vi "Dashboard Main.vi"() -> ()   [LabVIEW 2015]
uses:
  <vilib>/Utility/miscctls.llb/LVRowAndColumnTypeDef.ctl
  <vilib>/event_ctls.llb/eventvkey.ctl
  <vilib>/Rock Robotics/WPI/Dashboard/WPI_DashboardLogging Global.vi
  <vilib>/Rock Robotics/Network Tables/NT Read Numeric Array.vi
  <vilib>/Rock Robotics/Network Tables/NT Read Boolean.vi
  <vilib>/Rock Robotics/Network Tables/NT Write Boolean.vi
  <vilib>/Utility/config.llb/Write Key (String).vi
  <vilib>/Utility/config.llb/Write Key (I32).vi
  <vilib>/Utility/config.llb/NI_LVConfig.lvlib
panel:
  in  "TCP":refnum<k5>
  in  "Rec Mode":enum32{"Stop", "Record", "Playback"}(radio)
  in  "Vision":u16(ring) items=["Camera Off", "USB Camera SW", "USB Camera HW", "IP Camera"]
  out "Camera IP":string
  out "Image Message":string="Timeout in Camera Communications"
  in  "Dashboard Tab":T1(tab)
  in  "Select Auto":string(combo)
  out "NT Connection":bool
  in  "Camera Settings":T2={"Frame Rate"=30, "Compression"=30, "Size"=1} {"Frame Rate" scale=1.0..30.0; "Size" items=["640x480", "320x240", "160x120"]}
  out "MotorChart R":cluster{"Numeric":dbl, "Numeric":dbl}(graph)
  out "MotorChart L":T3(graph)
  out "MotorSliders R":cluster{"MotorSlide1":dbl, "MotorSlide2":dbl} {"MotorSlide2" scale=-1.0..1.0 scale format="%#_2e"; "MotorSlide1" scale=-1.0..1.0 scale format="%#_2e"}
  out "MotorSliders L":T4 {"MotorSlide4 2" scale=0.0..14.0 scale format="%#_2e"; "MotorSlide2" scale=-1.0..1.0 scale format="%#_2e"; "MotorSlide1" scale=-1.0..1.0 scale format="%#_2e"}
  out "Gyro":dbl(knob) scale=0.0..360.0
  out "JS1 Z":dbl(slide) scale=-1.0..1.0 scale format="%#_2e"
  out "JS1 Graph":cluster{"X":dbl, "Y":dbl}[](graph)
  out "JS1 Buttons":T5
  out "JS2 Z":dbl(slide) scale=-1.0..1.0 scale format="%#_2e"
  out "JS2 Graph":cluster{"X":dbl, "Y":dbl}[](graph)
  out "JS2 Buttons":T5
  out "Mode":T6(ring)=enum."Auto Disabled"
  in  "DB Camera Config":bool
  out "fps":dbl format="%#.1g"
  out "Mbps":dbl format="%#.1g"
  out "Mbps LED":bool
  in  "DB/String 9":string
  in  "DB/String 8":string
  in  "DB/String 7":string
  in  "DB/String 6":string
  in  "DB/String 5":string
  in  "DB/String 4":string
  in  "DB/String 3":string
  in  "DB/String 2":string
  in  "DB/String 1":string
  in  "DB/String 0":string
  in  "DB/Slider 0":dbl(slide) scale=0.0..5.0
  in  "DB/Slider 1":dbl(slide) scale=0.0..5.0
  in  "DB/Slider 2":dbl(slide) scale=0.0..5.0
  in  "DB/Slider 3":dbl(slide) scale=0.0..5.0
  out "DB/LED 3":bool
  out "DB/LED 2":bool
  out "DB/LED 1":bool
  out "DB/LED 0":bool
  in  "DB/Button 3":bool
  in  "DB/Button 2":bool
  in  "DB/Button 1":bool
  in  "DB/Button 0":bool caption="New Name"
  in  "Lower Shoot On Start of Auto":bool=TRUE
  in  "Auto Mode \nSelector":dbl
  out "?":dbl(slide)=88.0 scale=78.0..98.0
  out "POT Online?":bool
  out "?":dbl(knob)=87.99999517335185 scale=78.0..98.0
  out "True Solid Value":dbl=88.0
  out "POT Sensor":dbl(knob)=88.0000526149156 scale=78.0..98.0
  out "Low Sensor":bool=TRUE
  out "High Sensor":bool=TRUE
  in  "Test Slider":dbl(slide) scale=0.0..100.0 scale format="%#_3g"
  in  "On/Off":bool caption="Solenoid"
  in  "Test Name":u16(ring) items=["Select the test to run..."]
  in  "Test Tree":string(tree)
  in  "Motor":cluster{"Value":dbl, "Enable":bool} {"Value" scale=-1.0..1.0 scale format="%#_3g"}
  out "Progress":T7 {"Test Progress" scale=0.0..100.0}
  in  "Rev/Fwd":cluster{"Forward":bool, "Reverse":bool}
  in  "Test Ring":u16(ring) items=["Monochrome", "Color"]
  out "Cmd Status":string
  in  "Execute Command":bool
  in  "Command Params":string[][](table)
  in  "Command Selection":i32(listbox)
  in  "CheckList":i32(listbox)
  out "Tree":string(tree)
  out "Camera Image":T8(plugin-control)
  out "Background":bool
  # "Left"
  # "Front"
  # "Right"
  # "Battery"
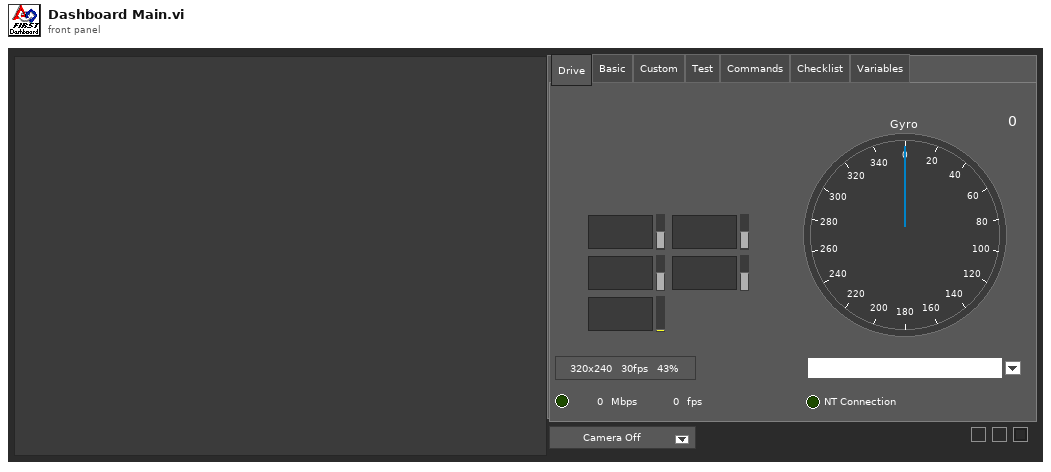
[diagram p1: front panel]
types:
  T1 = enum32{"Drive", "Basic", "Custom", "Test", "Commands", "Checklist", "Variables"}
  T2 = cluster{"Frame Rate":i32, "Compression":i32, "Size":u16}
  T3 = cluster{"Numeric":dbl, "Numeric":dbl, "Battery V":dbl}
  T4 = cluster{"MotorSlide1":dbl, "MotorSlide2":dbl, "MotorSlide4 2":dbl}
  T5 = cluster{bool, bool, bool, bool, bool, bool, bool, bool, bool, bool, bool, bool}
  T6 = enum8{"Tele-Op Disabled", "Tele-Op Enabled", "Auto Disabled", "Auto Enabled", "Test Disabled", "Test Enabled", "Disconnected", "No Code", "E-Stop"}
  T7 = cluster{"Test Progress":u8, "Test Progress Text":string}
  T8 = typedef "IMAQ Image.ctl" = refnum<image>
  T9 = cluster{"IDs":cluster{"RPC field ID":u16, "Unique ID":u16}, "String":string}
  T10 = enum32{"Drive", "Basic", "Custom", "Test", "Checklist", "Variables"}
  T11 = typedef "Image Type" = u32
  T12 = cluster{"Camera Image":refnum<vi>, "Dashboard Tab":refnum<vi>, "Background":refnum<vi>, "Vision":refnum<vi>, "Rec Mode":refnum<vi>, "Test Slider":refnum<vi>, "On/Off ":refnum<vi>, "Test Ring":refnum<vi>, "Rev/Fwd":refnum<vi>, "Test Name":refnum<vi>, "Motor":refnum<vi>, "Progress":refnum<vi>, "CheckList":refnum<vi>, "Tree":refnum<vi>, "Test Tree":refnum<vi>, "Command Params":refnum<vi>, "Command Selection":refnum<vi>, "Execute Command":refnum<vi>, "Cmd Status":refnum<vi>}
  T13 = cluster{"Error Strings":string, "Disable Counts":cluster{u16, u16}, "Rail Faults":cluster{u16, u16, u16}, "Robot IP":string, "DB Mode":u8, "Event Info":cluster{"Name":string, "Type":u8, "Number":u16, "Replay":u8}, "Camera Addr":string}
  T14 = cluster{"Storage":cluster{"Disk Free":u64, "RAM Block":u32, "RAM free":u32}, "CPU Utilization":cluster{"CPU % ISR":sgl, "CPU % Time Crit":sgl, "CPU % Timed Str":sgl, "CPU % High":sgl, "CPU % Above":sgl, "CPU % Normal":sgl, "CPU % Low":sgl}, "CAN":cluster{"% Bus Utilization":sgl, "Bus Off Cnt":u32, "TX_FIFO Full Cnt":u32, "Receive Error Cnt":u8, "Transmit Error Cnt":u8}, "HID":cluster{"HID Outputs":u32, "Rumble Low":u16, "Rumble High":u16}[]}
  T15 = cluster{"Status bits":cluster{"Test Mode":bool, "Autonomous":bool, "Enabled":bool, "Code Start":bool, "Brownout":bool, "Reserved 2":bool, "Reserved 3":bool, "E-Stop":bool}, "Code Trace":cluster{"Disabled":bool, "TeleOp":bool, "Auto":bool, "Test":bool}, "Controller Type":enum16{"unknown", "cRIO", "roboRio"}, "Code?":enum16{"unknown", "noCode", "code"}, "Battery V":dbl}
  T16 = cluster{"Control Bits":cluster{"TestMode":bool, "Autonomous":bool, "Enabled":bool, "FMS Present":bool, bool, bool, bool, "E-Stop":bool}, "Team Station ":u8, "Countdown":sgl, "Joystick Values":cluster{"Axes":dbl[], "Buttons":bool[], "POVs":i16[]}[]}
  T17 = cluster{"Axes":dbl[], "Buttons":bool[], "POVs":i16[]}[]
  T18 = cluster{"Axes":dbl[], "Buttons":bool[], "POVs":i16[]}
  T19 = cluster{"Buttons[0]":bool, "Buttons[1]":bool, "Buttons[2]":bool, "Buttons[3]":bool, "Buttons[4]":bool, "Buttons[5]":bool, "Buttons[6]":bool, "Buttons[7]":bool, "Buttons[8]":bool, "Buttons[9]":bool, "Buttons[10]":bool, "Buttons[11]":bool}
  T20 = typedef "NI_LVConfig.lvlib/Config Data RefNum.ctl" = refnum<k1>
  T21 = cluster{"Operation":enum16{"Update", "Clear"}, "Color Box":u32}[]
  T22 = typedef "eventvkey.ctl" = enum16{"ASCII", "Enter", "Return", "Shift", "Ctrl", "Alt", "Cmd", "Opt", "Caps", "NumLock", "Clear", "Break", "Up", "Down", "Left", "Right", "Insert", "Delete", "Home", "End", "PageUp", "PageDown", "Escape", "Help", "Pause", "ScrollLock", "F1", "F2", "F3", "F4", "F5", "F6", "F7", "F8", "F9", "F10", "F11", "F12", "F13", "F14", "F15", "F16", "F17", "F18", "F19", "F20", "F21", "F22", "F23", "F24", "Play", "VolumeUp", "VolumeDown", "Mute", "Two Byte Char"}
  T23 = cluster{"Image Size":bool, "Image Type":bool, "Pixel Value":bool, "ROI Information":bool, "Zoom Factor":bool}
  T24 = enum8{"Enabled", "Disabled", "Disabled and Grayed Out"}
  T25 = cluster{"Operation":enum16{"Update", "Clear"}, "Color Box":u32}
  T26 = typedef "LVRowAndColumnTypeDef.ctl" = cluster{"Row":i32, "Column":i32}
  T27 = cluster{"Shift":bool, "Ctrl":bool, "Alt":bool, "Cmd":bool, "Opt":bool}
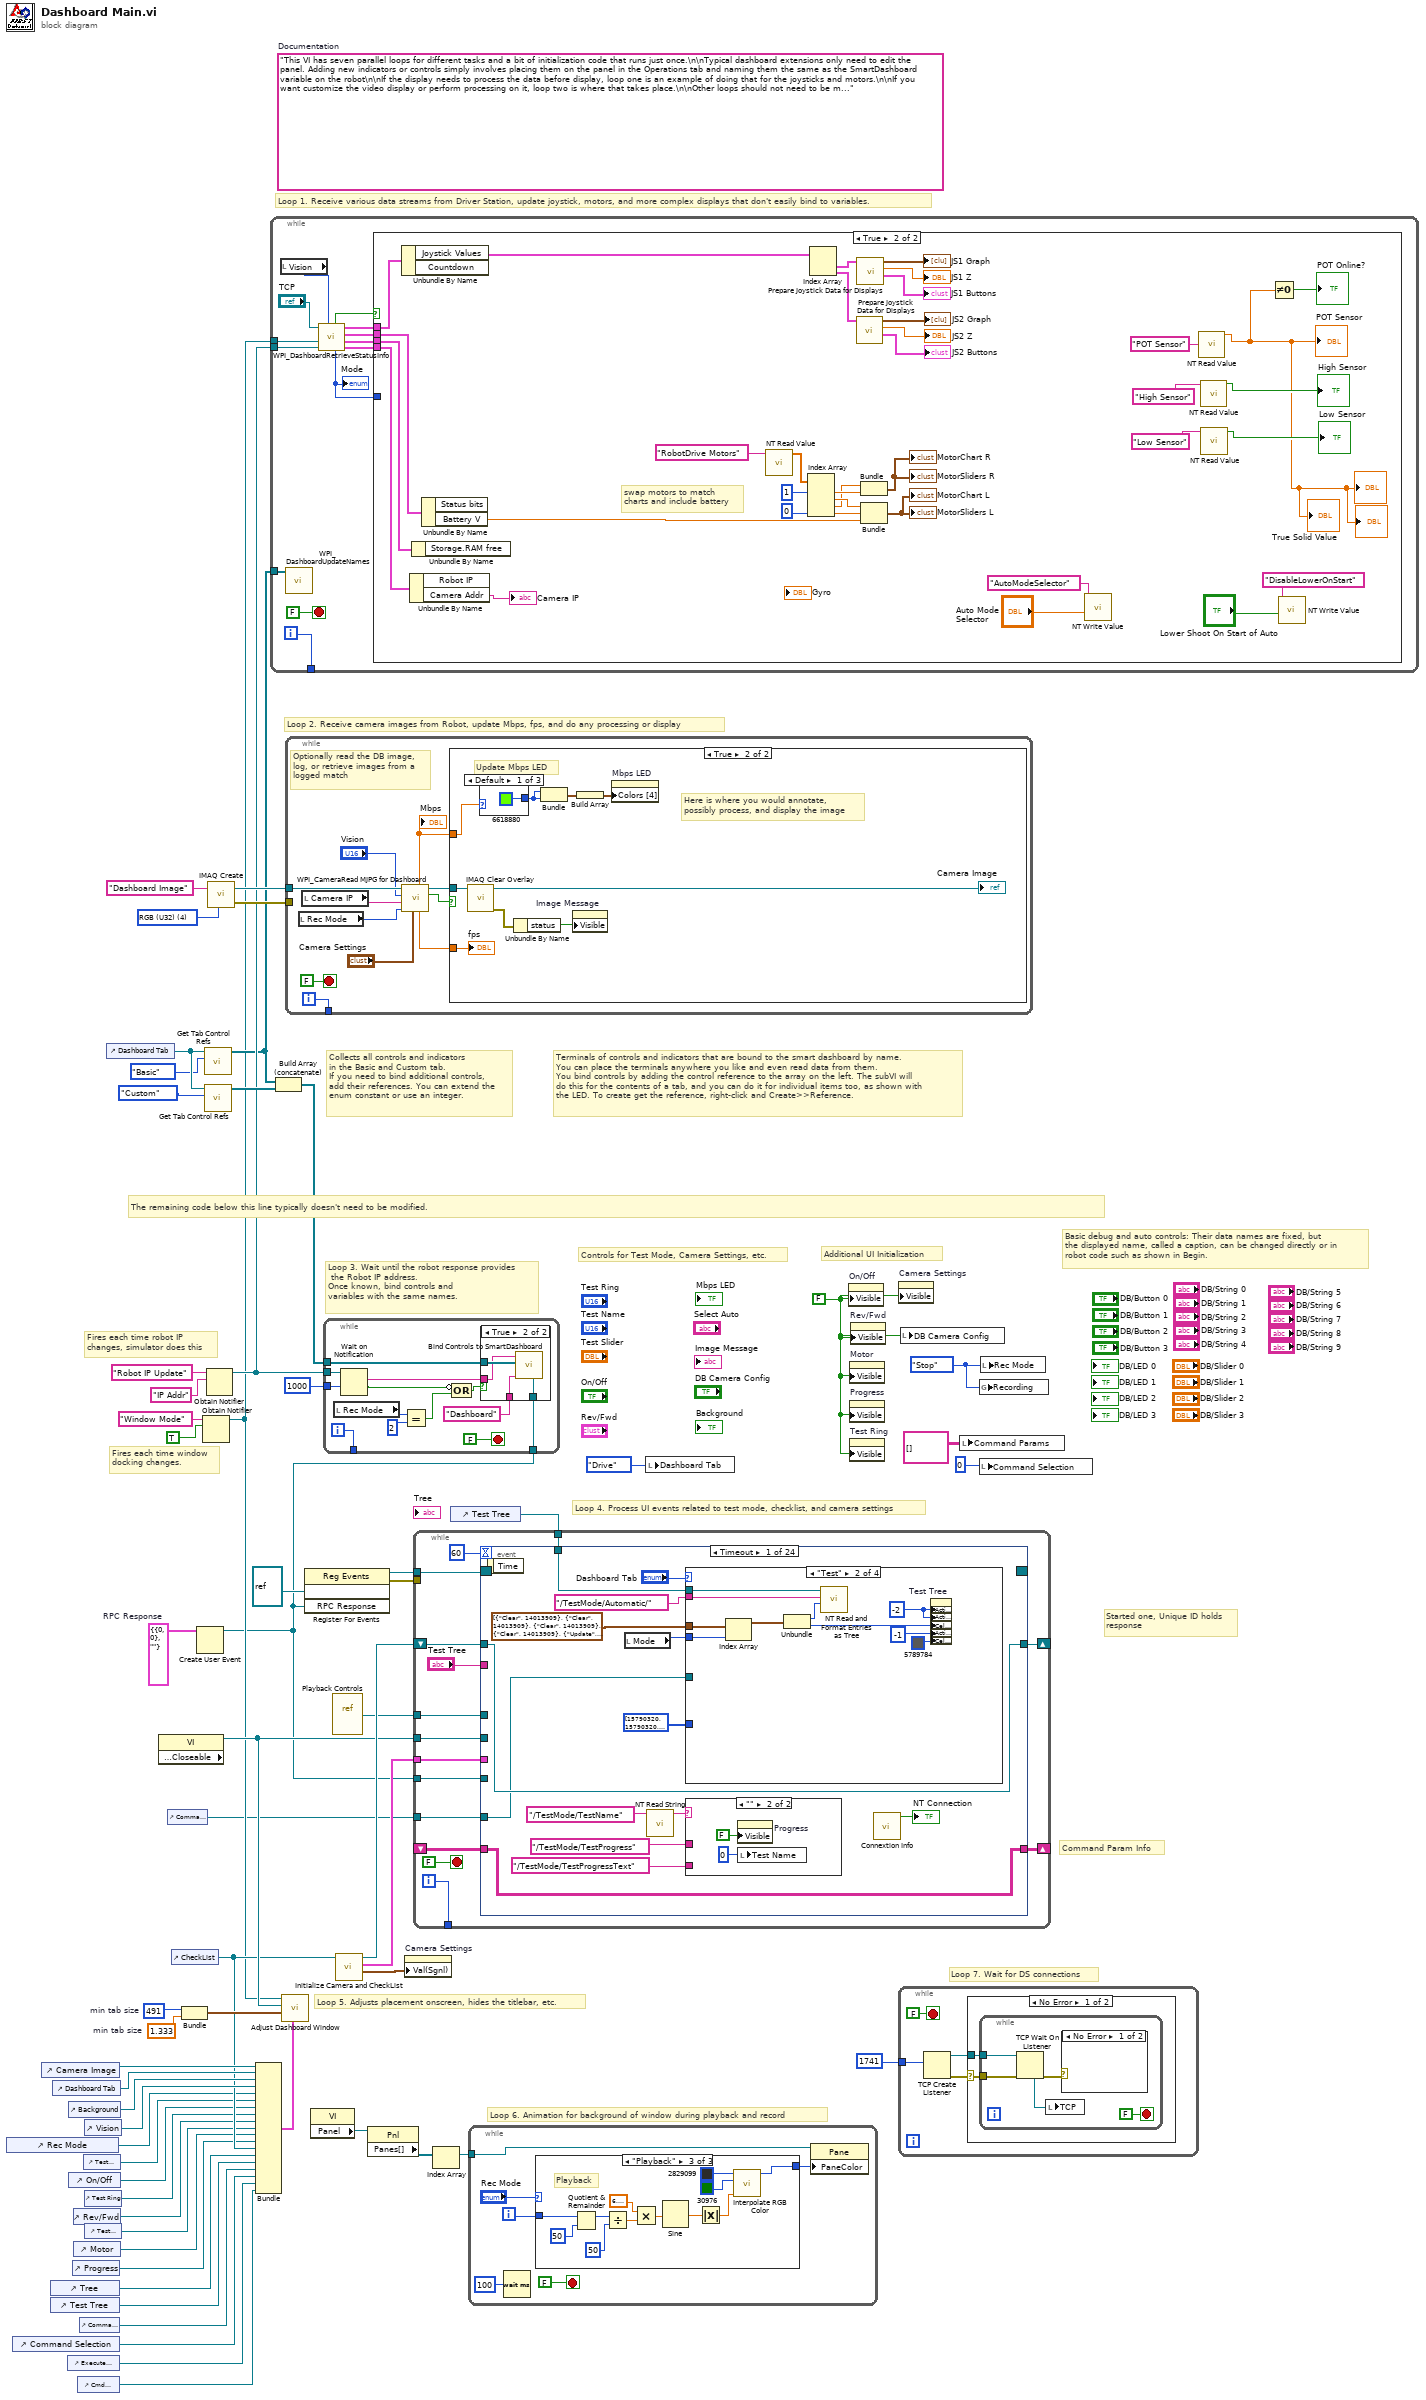
[diagram p0: block diagram]
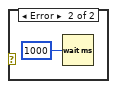
[diagram p2: hidden frame]
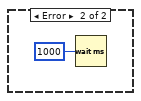
[diagram p3: hidden frame]
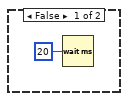
[diagram p4: hidden frame]
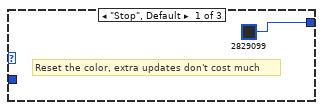
[diagram p5: hidden frame]
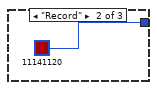
[diagram p6: hidden frame]
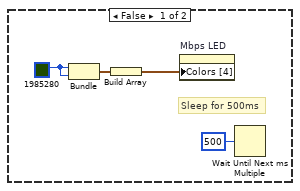
[diagram p8: hidden frame]
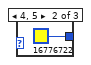
[diagram p9: hidden frame]
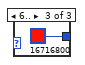
[diagram p10: hidden frame]
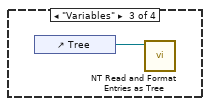
[diagram p12: hidden frame]
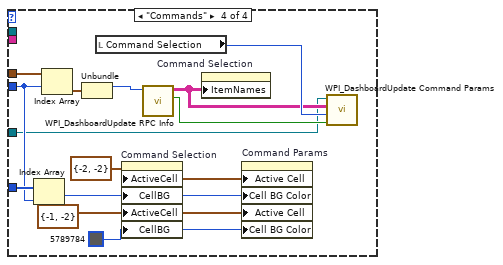
[diagram p13: hidden frame]
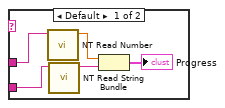
[diagram p14: hidden frame]
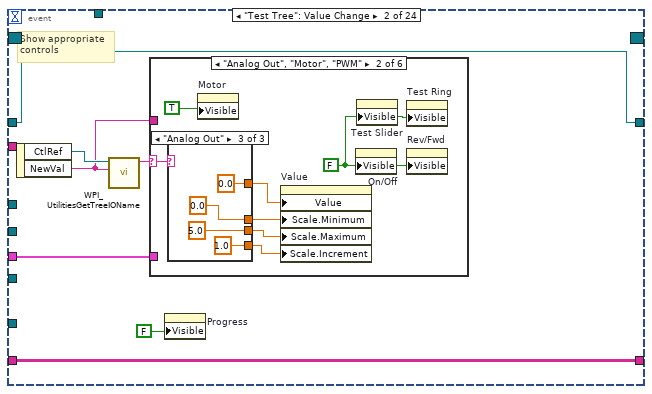
[diagram p15: hidden frame]
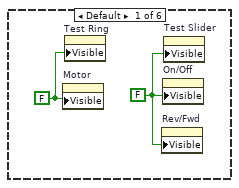
[diagram p16: hidden frame]
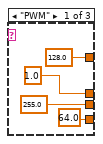
[diagram p17: hidden frame]
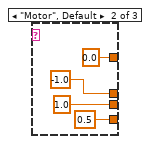
[diagram p18: hidden frame]
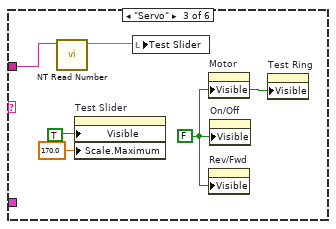
[diagram p19: hidden frame]
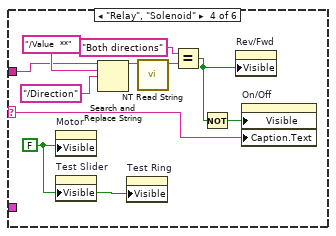
[diagram p20: hidden frame]
diagram:
  w7 = T9 {"IDs"={"RPC field ID"=0, "Unique ID"=0}, "String"=""}  # RPC Response
  w33 = 491  # min tab size
  w32 = 1.333  # min tab size
  w41 = enum32{"Stop", "Record", "Playback"}."Stop" ("Rec Mode")
  w15 = FALSE ("Visible")
  (unwired) "This VI has seven parallel loops for different tasks and a bit of initialization code that runs just once.\n\nTypical dashboard extensions only need to edit the panel. Adding new indicators or controls simply involves placing them on the panel in the Operations tab and naming them the same as the SmartDashboard variable on the robot\n\nIf the display needs to process the data before display, loop one is an example of doing that for the joysticks and motors.\n\nIf you want customize the video display or perform processing on it, loop two is where that takes place.\n\nOther loops should not need to be modified. They are pretty standard, and document the task they perform."  # Documentation
  w61 = T11 4 items=["Grayscale (U8)", "Grayscale (I16)", "Grayscale (SGL)", "Complex (CSG)", "RGB (U32)", "HSL (U32)", "RGB (U64)"] ("Image Type")
  # "Command Param Info"
  # "Started one, Unique ID holds\nresponse"
  # "Loop 7. Wait for DS connections"
  # "Basic debug and auto controls: Their data names are fixed, but\nthe displayed name, called a caption, can be changed directly or in\nrobot code such as shown in Begin."
  # "Controls for Test Mode, Camera Settings, etc."
  # "Additional UI Initialization"
  # "Loop 6. Animation for background of window during playback and record"
  # "Fires each time robot IP\nchanges, simulator does this"
  # "Fires each time window\ndocking changes."
  # "Collects all controls and indicators\nin the Basic and Custom tab.\nIf you need to bind additional controls,\nadd their references. You can extend the\nenum constant or use an integer."
  # "The remaining code below this line typically doesn't need to be modified."
  # "Loop 4. Process UI events related to test mode, checklist, and camera settings"
  # "Terminals of controls and indicators that are bound to the smart dashboard by name.\nYou can place the terminals anywhere you like and even read data from them.\nYou bind controls by adding the control reference to the array on the left. The subVI will\ndo this for the contents of a tab, and you can do it for individual items too, as shown with\nthe LED. To create get the reference, right-click and Create>>Reference."
  # "Loop 3. Wait until the robot response provides\n the Robot IP address.\nOnce known, bind controls and\nvariables with the same names."
  # "Loop 5. Adjusts placement onscreen, hides the titlebar, etc."
  # "Loop 1. Receive various data streams from Driver Station, update joystick, motors, and more complex displays that don't easily bind to variables."
  # "Loop 2. Receive camera images from Robot, update Mbps, fps, and do any processing or display"
  n1 = control-ref of="Rec Mode"() -> (w21:refnum<vi>)
  n2 = control-ref of="Command Selection"() -> (w6:refnum<vi>)
  n3 = control-ref of="Camera Image"() -> (w36:refnum<vi>)
  n4 = control-ref of="Tree"() -> (w25:refnum<vi>)
  n5 = control-ref of="Test Tree"() -> (w24:refnum<vi>)
  n6 = control-ref of="Dashboard Tab"() -> (w35:refnum<vi>)
  n7 = control-ref of="Execute Command"() -> (w8:refnum<vi>)
  n8 = control-ref of="Background"() -> (w30:refnum<vi>)
  n9 = control-ref of="On/Off"() -> (w19:refnum<vi>)
  n10 = control-ref of="Progress"() -> (w16:refnum<vi>)
  n11 = control-ref of="Rev/Fwd"() -> (w17:refnum<vi>)
  n12 = control-ref of="Motor"() -> (w22:refnum<vi>)
  n13 = control-ref of="Cmd Status"() -> (w2:refnum<vi>)
  n14 = control-ref of="Command Params"() -> (w9:refnum<vi>)
  n15 = control-ref of="Test Slider"() -> (w20:refnum<vi>)
  n16 = control-ref of="Vision"() -> (w34:refnum<vi>)
  n17 = control-ref of="Test Ring"() -> (w18:refnum<vi>)
  n18 = control-ref of="Test Name"() -> (w23:refnum<vi>)
  n19 = control-ref of="Dashboard Tab"() -> (w39:refnum<vi>)
  n20 = property class="VI" props=["Front Panel.Closeable"]() -> (reference out=w40:refnum<vi>)  [unwired: 2 in, 2 out]
  n21 = control-ref of="Command Params"() -> (w1:refnum<vi>)
  n22 = control-ref of="CheckList"() -> (w26:refnum<vi>)
  n23 = Bundle("min tab size"=w33, "min tab size"=w32) -> (w31:cluster{"min tab size":i32, "min tab size":dbl})  [unwired: 1 in]
  n24 = Create User Event(user event datatype=w7) -> (user event=w3:refnum<user-event>)  [unwired: 1 in, 1 out]
  n25 = Obtain Notifier(name (unnamed)="Window Mode", notification data type=TRUE) -> (notifier out=w12:refnum<notifier>)  [unwired: 2 in, 2 out]
  n26 = call <vilib>:"Get Tab Control Refs.vi"("Page Index"=T10."Basic" ("Dashboard Tab"), "TabControl in"=w39) -> ("ControlsOnPage"=w13:refnum<vi>[])  [unwired: 9 in]
  n27 = call <vilib>:"Get Tab Control Refs.vi"("Page Index"=T10."Custom" ("Dashboard Tab"), "TabControl in"=w39) -> ("ControlsOnPage"=w38:refnum<vi>[])  [unwired: 9 in]
  n28 = Obtain Notifier(name (unnamed)="Robot IP Update", notification data type="IP Addr" ("name (unnamed)")) -> (notifier out=w14:refnum<notifier>)  [unwired: 2 in, 2 out]
  n29 = call "IMAQ Create"("Image Name"="Dashboard Image", "Image Type"=w61) -> ("New Image"=w59:T8, "error out"=w58:errorcluster)  [unwired: 2 in, 1 out]
  n30 = Bundle("Camera Image"=w36, "Dashboard Tab"=w35, "Background"=w30, "Vision"=w34, "Rec Mode"=w21, "Test Slider"=w20, "On/Off"=w19, "Test Ring"=w18, "Rev/Fwd"=w17, "Test Name"=w23, "Motor"=w22, "Progress"=w16, "CheckList"=w26, "Tree"=w25, "Test Tree"=w24, "Command Params"=w9, "Command Selection"=w6, "Execute Command"=w8, "Cmd Status"=w2) -> (w27:T12)  [unwired: 1 in]
  n31 = while {
    tunnel: [w73] -> _
    tunnel: w14 -> [w67]
    tunnel: w13 -> [w66]
    tunnel: w12 -> [w62]
    i -> [w73]
    stop <- FALSE stop-if-true
    n32 = local read "Vision"() -> (w64:u16)
    n33 = call <vilib>:"WPI_DashboardUpdateNames.vi"("Controls on Tab"=w66) -> ()  [unwired: 11 in]
    n34 = call <vilib>:"WPI_DashboardRetrieveStatusInfo.vi"("Vision"=w64, "Binding Refnum"=w67, "Window Mode Notifier"=w62, "TCP Cnx"="TCP") -> ("Power and Errors"=w68:T13, "Robot Metrics"=w71:T14, "Status Info"=w72:T15, "Control Info"=w69:T16, "Robot Mode"=w65:T6, "Process?"=w70:bool)  [unwired: 2 in]
    "Mode" <- w65
    n35 = case shown="True" w70 {
      tunnel: w72 -> [_ w111]
      tunnel: w71 -> [_ w110]
      tunnel: w69 -> [_ w109]
      tunnel: w68 -> [_ w108]
      tunnel: w65 -> [_ _]
      frame False {
        n36 = Wait (ms)(milliseconds to wait=u32 20) -> ()  [unwired: 1 out]
      }
      frame True {
        # "swap motors to match\ncharts and include battery"
        n37 = Unbundle By Name(w109) -> ("Joystick Values"=w98:T17)  [unwired: 1 out]
        n38 = Unbundle By Name(w108) -> ("Camera Addr"=→"Camera IP":string)  [unwired: 1 out]
        n39 = Unbundle By Name(w110) -> ()  [unwired: 1 out]
        n40 = Unbundle By Name(w111) -> ("Battery V"=w99:dbl)  [unwired: 1 out]
        n41 = call-poly <vilib>:"NT Read Value.vi"("Name"="RobotDrive Motors") -> ("Numeric Array"=w87:dbl[])  [unwired: 9 in, 1 out]
        n42 = Index Array(array=w87, index #1=1, index #4=0) -> (element #1=w103:dbl, element #2=w104:dbl, element #3=w102:dbl, element #4=w107:dbl)  [unwired: 2 in]
        n43 = Index Array(array=w98) -> (element #1=w97:T18, element #2=w92:T18)  [unwired: 2 in]
        n44 = call "Prepare Joystick Data for Displays.vi"("Joystick Values"=w92) -> ("Buttons"=→"JS2 Buttons":T19, "Z Axis"=→"JS2 Z":dbl, "Cartesian Data"=→"JS2 Graph":cluster{"X axis":dbl, "X axis":dbl}[])  [unwired: 8 in]
        n45 = call "Prepare Joystick Data for Displays.vi"("Joystick Values"=w97) -> ("Buttons"=→"JS1 Buttons":T19, "Z Axis"=→"JS1 Z":dbl, "Cartesian Data"=→"JS1 Graph":cluster{"X axis":dbl, "X axis":dbl}[])  [unwired: 8 in]
        n46 = Bundle("Numeric"=w102, "Numeric"=w103) -> (→"MotorChart R" →"MotorSliders R":cluster{"Numeric":dbl, "Numeric":dbl})  [unwired: 1 in]
        n47 = Bundle("Numeric"=w104, "Numeric"=w107, "Battery V"=w99) -> (→"MotorChart L" →"MotorSliders L":T3)  [unwired: 1 in]
        n48 = call-poly <vilib>:"NT Write Value.vi"("Numeric"="Auto Mode \nSelector", "Name"="AutoModeSelector") -> ()  [unwired: 9 in, 1 out]
        n49 = call-poly <vilib>:"NT Read Value.vi"("Name"="POT Sensor") -> ("Numeric"=w76:dbl)  [unwired: 9 in, 1 out]
        "POT Sensor" <- w76
        "True Solid Value" <- w76
        "?" <- w76
        "?" <- w76
        n50 = call-poly <vilib>:"NT Read Value.vi"("Name"="High Sensor") -> ("Boolean"=→"High Sensor":bool)  [unwired: 9 in, 1 out]
        n51 = call-poly <vilib>:"NT Read Value.vi"("Name"="Low Sensor") -> ("Boolean"=→"Low Sensor":bool)  [unwired: 9 in, 1 out]
        n52 = Not Equal To 0?(x=w76) -> (x != 0?=→"POT Online?":bool)
        n53 = call-poly <vilib>:"NT Write Value.vi"("Boolean"="Lower Shoot On Start of Auto", "Name"="DisableLowerOnStart") -> ()  [unwired: 9 in, 1 out]
      }
    }
  }
  n54 = Build Array (concatenate)(w13, w38) -> (w37:refnum<vi>[])
  n55 = call "Adjust Dashboard Window.vi"("Sizing Refnums"=w27, "Size Constraints"=w31, "VI"=w40, "WIn Mode"=w12) -> ()  [unwired: 8 in]
  n56 = while {
    tunnel: w59 -> [w120]
    tunnel: w58 -> [_]
    tunnel: [w121] -> _
    i -> [w121]
    stop <- FALSE stop-if-true
    # "Optionally read the DB image,\nlog, or retrieve images from a\nlogged match"
    n57 = local read "Rec Mode"() -> (w115:enum32{"Stop", "Record", "Playback"})
    n58 = local read "Camera IP"() -> (w113:string)
    n59 = call <vilib>:"WPI_CameraRead MJPG for Dashboard.vi"("Camera Settings"="Camera Settings", "Rec Mode"=w115, "Camera IP"=w113, "Camera Mode"="Vision", "Refnum in"=w120) -> ("Active"=w118:bool, "Refnum out"=w119:T8, "FPS"=w117:dbl, "Bandwidth (Mbps)"=w112:dbl)  [unwired: 3 in]
    "Mbps" <- w112
    n60 = case shown="True" w118 {
      tunnel: w119 -> [_ w130]
      tunnel: w112 -> [_ w129]
      tunnel: w117 -> [_ w127]
      frame False {
        w123 = u32 1985280 ("Color Box")
        # "Sleep for 500ms"
        n61 = Bundle("Color Box"=w123, "Color Box"=w123) -> (w125:cluster{"Color Box":u32, "Color Box":u32})  [unwired: 1 out]
        n62 = Build Array(w125) -> (w124:cluster{"Color Box":u32, "Color Box":u32}[])
        n63 = property on="Mbps LED" class="Bool (strict)"("Colors [4]"=w124) -> ()  [unwired: 2 in, 2 out]
        n64 = Wait Until Next ms Multiple(millisecond multiple=u32 500) -> ()  [unwired: 1 out]
      }
      frame True {
        # "Here is where you would annotate,\npossibly process, and display the image"
        # "Update Mbps LED"
        n65 = call "IMAQ Clear Overlay"("Image"=w130) -> ("error out"=w134:errorcluster, "Image Out"=→"Camera Image":T8)  [unwired: 2 in, 7 out]
        n66 = case shown="Default" w129 {
          tunnel: [u32 6618880 ("Color Box") u32 16776722 ("Color Box") u32 16716800 ("Color Box")] -> w131
          frame Default {
          }
          frame 4, 5 {
          }
          frame 6.. {
          }
        }
        n67 = Unbundle By Name(w134) -> ("status"=w135:bool)
        n68 = Bundle("Color Box"=w131, "Color Box"=w131) -> (w133:cluster{"Color Box":u32, "Color Box":u32})  [unwired: 1 out]
        n69 = property on="Image Message" class="Str"("Visible"=w135) -> ()  [unwired: 2 in, 2 out]
        n70 = Build Array(w133) -> (w132:cluster{"Color Box":u32, "Color Box":u32}[])
        n71 = property on="Mbps LED" class="Bool (strict)"("Colors [4]"=w132) -> ()  [unwired: 2 in, 2 out]
        "fps" <- w127
      }
    }
  }
  n72 = register-events(refnum<vi> refnum, w3) -> (reference out=w45:refnum<event-registration>, error out=w44:errorcluster)  [unwired: 2 in]
  n73 = property class="VI"() -> ("Panel"=w48:refnum<vi>)  [unwired: 2 in, 2 out]
  n74 = while {
    tunnel: w37 -> [w151]
    tunnel: w14 -> [w149]
    tunnel: [w147] -> _
    tunnel: u32 1000 ("milliseconds to wait") -> [w146]
    tunnel: w3 -> [w139]
    i -> [w147]
    stop <- FALSE stop-if-true
    n75 = local read "Rec Mode"() -> (w142:enum32{"Stop", "Record", "Playback"})
    n76 = Wait on Notification(notifier=w149, timeout in ms (-1)=w146) -> (notification=w148:string, timed out?=w144:bool)  [unwired: 2 in, 2 out]
    n77 = Equal?(x=w142, y=u16 2 ("Rec Mode")) -> (x = y?=w143:bool)
    n78 = Compound Arithmetic op=OR(invert w144, w143) -> (w145:bool)
    n79 = case shown="True" w145 {
      tunnel: w151 -> [_ w155]
      tunnel: w148 -> [_ w154]
      tunnel: "Dashboard" -> [_ w153]
      tunnel: w139 -> [_ w152]
      frame False {
      }
      frame True {
        n80 = call <vilib>:"Bind Controls to SmartDashboard.vi"("RPC ref"=w152, "Client Name"=w153, "Bound Control Refs"=w155, "Server IP Address"=w154) -> ()  [unwired: 8 in]
      }
    }
  }
  n81 = vi-ref "Playback Controls.vi"() -> (w46:refnum<vi>)
  n82 = call "Initialize Camera and CheckList.vi"("ListBox in"=w26) -> ("Cluster"=w52:cluster{"value":i32, "value":i32, "index":i32}, "Array"=w53:cluster{string[]}[], "File Refnum"=w51:T20)  [unwired: 8 in]
  n83 = property class="Pnl"(reference=w48) -> ("Panes[]"=w49:refnum<vi>[])  [unwired: 1 in, 2 out]
  n84 = property on="Camera Settings" class="Clust (strict)"("Val(Sgnl)"=w52) -> ()  [unwired: 2 in, 2 out]
  n85 = Index Array(array=w49) -> (element=w47:refnum<vi>)  [unwired: 1 in]
  n86 = control-ref of="Test Tree"() -> (w50:refnum<vi>)
  n87 = while {
    tunnel: w53 -> [w167]
    shift-right: [w166] -> _
    shift-left: w51 -> [w165]
    tunnel: [w164] -> _
    tunnel: w50 -> [w163]
    tunnel: w46 -> [w162]
    tunnel: w45 -> [w161]
    tunnel: w44 -> [_]
    tunnel: w40 -> [w160]
    tunnel: w3 -> [w159]
    tunnel: w1 -> [w158]
    shift-right: [w157] -> _
    shift-left: _ -> [w156]
    i -> [w164]
    stop <- FALSE stop-if-true
    n88 = event shown="[0] Timeout" {
      selector: w161 -> [_ _ _ _ _ _ _ _ _ _ _ _ _ _ _ _ _ _ _ _ _ _ _ _]
      dyn-events: [_ _ _ _ _ _ _ _ _ _ _ _ _ _ _ _ _ _ w476 _ _ _ _ _] -> _
      timeout: u32 60 ("milliseconds to wait") -> [_ _ _ _ _ _ _ _ _ _ _ _ _ _ _ _ _ _ _ _ _ _ _ _]
      tunnel: w163 -> [w180 _ _ _ _ _ _ _ _ _ _ _ _ _ _ _ _ _ _ _ _ _ _ _]
      tunnel: "Test Tree" -> [_ _ _ _ _ _ _ _ _ _ _ _ _ w439 w448 w451 w456 w465 _ _ _ _ _ _]
      tunnel: w167 -> [_ w218 _ _ _ _ _ _ _ _ _ w401 w432 _ _ _ _ _ _ _ _ _ _ _]
      tunnel: [w177 w217 w321 w327 w337 w341 w347 w359 w367 w373 w386 w400 w425 w438 w446 w450 w455 w464 w478 w494 w496 w504 w515 w520] -> w166
      tunnel: w165 -> [w177 w217 w321 w327 w337 w341 w347 w359 w367 w373 w386 w399 w425 w438 w446 w450 w455 w464 w478 w494 w496 w504 w515 w520]
      tunnel: w162 -> [_ _ _ _ _ _ _ _ _ _ _ _ _ _ _ _ _ _ w479 _ w499 _ _ _]
      tunnel: w160 -> [_ _ _ _ _ _ _ _ _ _ _ _ _ _ _ _ _ _ w474 _ _ _ _ _]
      tunnel: w159 -> [_ _ _ _ _ _ _ _ _ _ _ _ _ _ _ _ _ _ w470 _ _ _ _ _]
      tunnel: w158 -> [w172 _ _ _ _ _ w345 _ _ _ _ _ _ _ _ _ _ _ _ _ _ _ _ _]
      tunnel: [w171 w216 w320 w326 w336 w342 w343 w353 w364 w372 w385 w398 w424 w437 w445 w449 w454 w463 w469 w492 w495 w500 w508 w521] -> w157
      tunnel: w156 -> [w171 w216 w320 w326 w336 w342 w343 _ _ w372 w385 w398 w424 w437 w445 w449 w454 w463 w469 w492 w495 w500 w508 w521]
      event Timeout {
        n89 = event-data() -> ()  [unwired: 1 in, 1 out]
        n90 = local read "Mode"() -> (w174:T6)
        n91 = call <vilib>:"NT Read String.vi"("Name"="/TestMode/TestName") -> ("String"=w183:string)  [unwired: 9 in, 1 out]
        n92 = case shown="\"Test\"" "Dashboard Tab" {
          tunnel: w180 -> [_ w194 _ _]
          tunnel: "/TestMode/Automatic/" ("Name Pattern") -> [_ w193 _ _]
          tunnel: T21 [{"Operation"=enum."Clear", "Color Box"=14013909}, {"Operation"=enum."Clear", "Color Box"=14013909}, {"Operation"=enum."Clear", "Color Box"=14013909}, {"Operation"=enum."Clear", "Color Box"=14013909}, {"Operation"=enum."Update", "Color Box"=14013909}, {"Operation"=enum."Update", "Color Box"=16777215}, {"Operation"=enum."Clear", "Color Box"=14013909}, {"Operation"=enum."Clear", "Color Box"=14013909}, {"Operation"=enum."Clear", "Color Box"=14013909}] -> [_ w186 _ w203]
          tunnel: w174 -> [_ w185 _ w202]
          tunnel: u32[] [15790320, 15790320, 15790320, 15790320, 16777215, 16777215, 15790320, 15790320, 15790320] -> [_ _ _ w208]
          tunnel: w172 -> [_ _ _ w196]
          frame "Custom", Default {
          }
          frame "Test" {
            w192 = -2 ("Active Item:Row Number")
            n93 = Index Array(array=w186, index=w185) -> (element=w187:T25)
            n94 = Unbundle(w187) -> ("Operation"=w188:enum16{"Update", "Clear"}, "Color Box"=w189:u32)
            n95 = call <vilib>:"NT Read and Format Entries as Tree.vi"("Operation"=w188, "Name Pattern"=w193, "Tree Refnum"=w194) -> ()  [unwired: 7 in, 2 out]
            n96 = property on="Test Tree" class="Tree (strict)"("Active Item Row Number"=w192, "ActiveColNum"=w192, "CellBG"=w189, "Active Item Row Number"=-1 ("Active Item:Row Number"), "CellBG"=u32 5789784 ("Color Box")) -> ()  [unwired: 2 in, 2 out]
          }
          frame "Variables" {
            n97 = control-ref of="Tree"() -> (w195:refnum<vi>)
            n98 = call <vilib>:"NT Read and Format Entries as Tree.vi"("Tree Refnum"=w195) -> ()  [unwired: 9 in, 2 out]
          }
          frame "Commands" {
            w204 = u32 5789784 ("Color Box")
            w205 = T26 {"Row"=-1, "Column"=-2} ("Active Cell:Active Cell")
            w207 = T26 {"Row"=-2, "Column"=-2} ("Active Cell:Active Cell")
            n99 = Index Array(array=w208, index=w202) -> (element=w206:u32)
            n100 = Index Array(array=w203, index=w202) -> (element=w201:T25)
            n101 = Unbundle(w201) -> ("Operation"=w200:enum16{"Update", "Clear"})  [unwired: 1 out]
            n102 = local read "Command Selection"() -> (w199:i32)
            n103 = property on="Command Selection" class="MCListbox (strict)"("ActiveCell"=w207, "CellBG"=w206, "ActiveCell"=w205, "CellBG"=w204) -> ()  [unwired: 2 in, 2 out]
            n104 = call <vilib>:"WPI_DashboardUpdate RPC Info.vi"("Operation"=w200) -> ("update"=w198:bool, "commands"=w197:string[][])  [unwired: 9 in]
            n105 = property on="Command Selection" class="MCListbox (strict)"("ItemNames"=w197) -> ()  [unwired: 2 in, 2 out]
            n106 = property on="Command Params" class="Tbl (strict)"("Active Cell"=w207, "Cell BG Color"=w206, "Active Cell"=w205, "Cell BG Color"=w204) -> ()  [unwired: 2 in, 2 out]
            n107 = call <vilib>:"WPI_DashboardUpdate Command Params.vi"("Update"=w198, "NewVal"=w199, "Commands"=w197, "Param Tbl"=w196) -> ()  [unwired: 7 in, 1 out]
          }
        }
        n108 = case shown="\"\"" w183 {
          tunnel: "/TestMode/TestProgress" ("Name") -> [w210 _]
          tunnel: "/TestMode/TestProgressText" ("Name") -> [w209 _]
          frame Default {
            n109 = call <vilib>:"NT Read Number.vi"("Name"=w210) -> ("Numeric"=w211:dbl)  [unwired: 9 in, 1 out]
            n110 = call <vilib>:"NT Read String.vi"("Name"=w209) -> ("String"=w212:string)  [unwired: 9 in, 1 out]
            n111 = Bundle("Numeric"=w211, "String"=w212) -> (→"Progress":cluster{"Numeric":dbl, "String":string})  [unwired: 1 in]
          }
          frame "" {
            n112 = property on="Progress" class="Clust (strict)"("Visible"=FALSE) -> ()  [unwired: 2 in, 2 out]
            n113 = local write "Test Name"(u16 0) -> ()
          }
        }
        n114 = call <vilib>:"Connextion Info.vi"() -> ("Connected"=→"NT Connection":bool)  [unwired: 10 in, 1 out]
      }
      event "Test Tree": Value Change {
        # "Show appropriate\ncontrols"
        n115 = event-data() -> ("CtlRef"=w221:refnum<vi>, "NewVal"=w219:string)  [unwired: 1 in]
        n116 = call <vilib>:"WPI_UtilitiesGetTreeIOName.vi"("NewVal"=w219, "TreeControl in"=w221) -> ("I/O Name"=w222:string)  [unwired: 9 in]
        n117 = case shown="\"Analog Out\", \"Motor\", \"PWM\"" w222 {
          selector: w222 -> [_ w229 _ w251 w260 _]
          tunnel: w219 -> [_ _ w248 w250 _ w267]
          tunnel: w218 -> [_ _ _ _ _ w266]
          frame Default {
            w224 = FALSE ("Visible")
            w223 = FALSE ("Visible")
            n118 = property on="Motor" class="Clust (strict)"("Visible"=w223) -> ()  [unwired: 2 in, 2 out]
            n119 = property on="Test Ring" class="Ring (strict)"("Visible"=w223) -> ()  [unwired: 2 in, 2 out]
            n120 = property on="Rev/Fwd" class="Clust (strict)"("Visible"=w224) -> ()  [unwired: 2 in, 2 out]
            n121 = property on="On/Off" class="Bool (strict)"("Visible"=w224) -> ()  [unwired: 2 in, 2 out]
            n122 = property on="Test Slider" class="Slide (strict)"("Visible"=w224) -> ()  [unwired: 2 in, 2 out]
          }
          frame "Analog Out", "Motor", "PWM" {
            w230 = FALSE ("Visible")
            n123 = case shown="\"Analog Out\"" w229 {
              tunnel: [1.0 ("Value") -1.0 ("Value") 0.0 ("Value")] -> w228
              tunnel: [255.0 ("Value") 1.0 ("Value") 5.0 ("Value")] -> w227
              tunnel: [128.0 ("Value") 0.0 ("Value") 0.0 ("Value")] -> w226
              tunnel: [64.0 ("Value") 0.5 ("Value") 1.0 ("Value")] -> w225
              frame "PWM" {
              }
              frame "Motor", Default {
              }
              frame "Analog Out" {
              }
            }
            n124 = property on="Motor" class="Clust (strict)"("Visible"=TRUE) -> ()  [unwired: 2 in, 2 out]
            n125 = property on="Value" class="Slide (strict)"("Value"=w226, "Scale.Minimum"=w228, "Scale.Maximum"=w227, "Scale.Increment"=w225) -> ()  [unwired: 2 in, 2 out]
            n126 = property on="On/Off" class="Bool (strict)"("Visible"=w230) -> ()  [unwired: 2 in, 2 out]
            n127 = property on="Test Slider" class="Slide (strict)"("Visible"=w230) -> ()  [unwired: 2 in, 2 out]
            n128 = property on="Test Ring" class="Ring (strict)"("Visible"=w230) -> ()  [unwired: 2 in, 2 out]
            n129 = property on="Rev/Fwd" class="Clust (strict)"("Visible"=w230) -> ()  [unwired: 2 in, 2 out]
          }
          frame "Servo" {
            w246 = FALSE ("Visible")
            n130 = call <vilib>:"NT Read Number.vi"("Name"=w248) -> ("Numeric"=w247:dbl)  [unwired: 9 in, 1 out]
            n131 = property on="Test Slider" class="Slide (strict)"("Visible"=TRUE, "Scale.Maximum"=170.0 ("Scale.Range:Maximum")) -> ()  [unwired: 2 in, 2 out]
            n132 = local write "Test Slider"(w247) -> ()
            n133 = property on="Motor" class="Clust (strict)"("Visible"=w246) -> ()  [unwired: 2 in, 2 out]
            n134 = property on="Rev/Fwd" class="Clust (strict)"("Visible"=w246) -> ()  [unwired: 2 in, 2 out]
            n135 = property on="On/Off" class="Bool (strict)"("Visible"=w246) -> ()  [unwired: 2 in, 2 out]
            n136 = property on="Test Ring" class="Ring (strict)"("Visible"=w246) -> ()  [unwired: 2 in, 2 out]
          }
          frame "Relay", "Solenoid" {
            w249 = FALSE ("Visible")
            n137 = property on="Motor" class="Clust (strict)"("Visible"=w249) -> ()  [unwired: 2 in, 2 out]
            n138 = property on="Test Slider" class="Slide (strict)"("Visible"=w249) -> ()  [unwired: 2 in, 2 out]
            n139 = Search and Replace String(input string=w250, search string="/Value  **", replace string="/Direction") -> (result string=w256:string)  [unwired: 5 in, 3 out]
            n140 = property on="Test Ring" class="Ring (strict)"("Visible"=w249) -> ()  [unwired: 2 in, 2 out]
            n141 = call <vilib>:"NT Read String.vi"("Name"=w256) -> ("String"=w254:string)  [unwired: 9 in, 1 out]
            n142 = Equal?(x="Both directions", y=w254) -> (x = y?=w252:bool)
            n143 = Not(x=w252) -> (.not. x?=w253:bool)
            n144 = property on="Rev/Fwd" class="Clust (strict)"("Visible"=w252) -> ()  [unwired: 2 in, 2 out]
            n145 = property on="On/Off" class="Bool (strict)"("Visible"=w253, "Caption.Text"=w251) -> ()  [unwired: 2 in, 2 out]
          }
          frame "Compressor", "Digital Out" {
            w259 = FALSE ("Visible")
            # "Get direction and finish"
            n146 = property on="Motor" class="Clust (strict)"("Visible"=w259) -> ()  [unwired: 2 in, 2 out]
            n147 = property on="Test Slider" class="Slide (strict)"("Visible"=w259) -> ()  [unwired: 2 in, 2 out]
            n148 = property on="Test Ring" class="Ring (strict)"("Visible"=w259) -> ()  [unwired: 2 in, 2 out]
            n149 = property on="On/Off" class="Bool (strict)"("Visible"=TRUE, "Caption.Text"=w260) -> ()  [unwired: 2 in, 2 out]
            n150 = property on="Rev/Fwd" class="Clust (strict)"("Visible"=FALSE) -> ()  [unwired: 2 in, 2 out]
          }
          frame "Camera" {
            n151 = call <vilib>:"Get Last Path Segment.vi"("String in"=w267) -> ("String out"=w268:string)  [unwired: 10 in]
            n152 = property on="On/Off" class="Bool (strict)"("Visible"=FALSE) -> ()  [unwired: 2 in, 2 out]
            n153 = property on="Motor" class="Clust (strict)"("Visible"=FALSE) -> ()  [unwired: 2 in, 2 out]
            n154 = property on="Rev/Fwd" class="Clust (strict)"("Visible"=FALSE) -> ()  [unwired: 2 in, 2 out]
            n155 = case shown="\"White Balance  **\"" w268 {
              tunnel: w267 -> [w274 w283 w292 w301 w310 _ w316]
              tunnel: w266 -> [w272 w280 w289 w298 w307 _ _]
              frame "Size  **" {
                n156 = Index Array(array=w272) -> (element=w271:cluster{string[]})  [unwired: 1 in]
                n157 = call <vilib>:"NT Read String.vi"("Name"=w274) -> ("String"=w273:string)  [unwired: 9 in, 1 out]
                n158 = Unbundle(w271) -> (w269:string[])
                n159 = Match First String(2:w269, 3:w273) -> (0:w270:i32)  [unwired: 1 out]
                n160 = property on="Test Ring" class="Ring (strict)"("Value"=w270, "Strings []"=w269) -> ()  [unwired: 2 in, 2 out]
                n161 = property on="Test Ring" class="Ring (strict)"("Visible"=TRUE) -> ()  [unwired: 2 in, 2 out]
                n162 = property on="Test Slider" class="Slide (strict)"("Visible"=FALSE) -> ()  [unwired: 2 in, 2 out]
              }
              frame "White Balance  **" {
                n163 = Index Array(array=w280, index=1) -> (element=w281:cluster{string[]})
                n164 = call <vilib>:"NT Read String.vi"("Name"=w283) -> ("String"=w282:string)  [unwired: 9 in, 1 out]
                n165 = Unbundle(w281) -> (w278:string[])
                n166 = Match First String(2:w278, 3:w282) -> (0:w277:i32)  [unwired: 1 out]
                n167 = property on="Test Ring" class="Ring (strict)"("Value"=w277, "Strings []"=w278) -> ()  [unwired: 2 in, 2 out]
                n168 = property on="Test Ring" class="Ring (strict)"("Visible"=TRUE) -> ()  [unwired: 2 in, 2 out]
                n169 = property on="Test Slider" class="Slide (strict)"("Visible"=FALSE) -> ()  [unwired: 2 in, 2 out]
              }
              frame "Exposure  **" {
                n170 = Index Array(array=w289, index=2) -> (element=w290:cluster{string[]})
                n171 = call <vilib>:"NT Read String.vi"("Name"=w292) -> ("String"=w291:string)  [unwired: 9 in, 1 out]
                n172 = Unbundle(w290) -> (w286:string[])
                n173 = Match First String(2:w286, 3:w291) -> (0:w287:i32)  [unwired: 1 out]
                n174 = property on="Test Ring" class="Ring (strict)"("Value"=w287, "Strings []"=w286) -> ()  [unwired: 2 in, 2 out]
                n175 = property on="Test Ring" class="Ring (strict)"("Visible"=TRUE) -> ()  [unwired: 2 in, 2 out]
                n176 = property on="Test Slider" class="Slide (strict)"("Visible"=FALSE) -> ()  [unwired: 2 in, 2 out]
              }
              frame "Exposure Priority  **" {
                n177 = Index Array(array=w298, index=3) -> (element=w299:cluster{string[]})
                n178 = call <vilib>:"NT Read String.vi"("Name"=w301) -> ("String"=w300:string)  [unwired: 9 in, 1 out]
                n179 = Unbundle(w299) -> (w295:string[])
                n180 = Match First String(2:w295, 3:w300) -> (0:w296:i32)  [unwired: 1 out]
                n181 = property on="Test Ring" class="Ring (strict)"("Value"=w296, "Strings []"=w295) -> ()  [unwired: 2 in, 2 out]
                n182 = property on="Test Ring" class="Ring (strict)"("Visible"=TRUE) -> ()  [unwired: 2 in, 2 out]
                n183 = property on="Test Slider" class="Slide (strict)"("Visible"=FALSE) -> ()  [unwired: 2 in, 2 out]
              }
              frame "Color Enable  **" {
                n184 = Index Array(array=w307, index=4) -> (element=w308:cluster{string[]})
                n185 = call <vilib>:"NT Read String.vi"("Name"=w310) -> ("String"=w309:string)  [unwired: 9 in, 1 out]
                n186 = Unbundle(w308) -> (w304:string[])
                n187 = Match First String(2:w304, 3:w309) -> (0:w305:i32)  [unwired: 1 out]
                n188 = property on="Test Ring" class="Ring (strict)"("Value"=w305, "Strings []"=w304) -> ()  [unwired: 2 in, 2 out]
                n189 = property on="Test Ring" class="Ring (strict)"("Visible"=TRUE) -> ()  [unwired: 2 in, 2 out]
                n190 = property on="Test Slider" class="Slide (strict)"("Visible"=FALSE) -> ()  [unwired: 2 in, 2 out]
              }
              frame Default {
                n191 = property on="Test Ring" class="Ring (strict)"("Visible"=FALSE) -> ()  [unwired: 2 in, 2 out]
                n192 = property on="Test Slider" class="Slide (strict)"("Visible"=FALSE) -> ()  [unwired: 2 in, 2 out]
              }
              frame "Brightness  **", "Color Level  **", "Compression  **", "FPS  **", "Sharpness  **" {
                n193 = call <vilib>:"NT Read Number.vi"("Name"=w316) -> ("Numeric"=w315:dbl)  [unwired: 9 in, 1 out]
                n194 = local write "Test Slider"(w315) -> ()
                n195 = property on="Test Slider" class="Slide (strict)"("Visible"=TRUE, "Scale.Maximum"=100.0 ("Scale.Range:Maximum")) -> ()  [unwired: 2 in, 2 out]
                n196 = property on="Test Ring" class="Ring (strict)"("Visible"=FALSE) -> ()  [unwired: 2 in, 2 out]
              }
            }
          }
        }
        n197 = property on="Progress" class="Clust (strict)"("Visible"=FALSE) -> ()  [unwired: 2 in, 2 out]
      }
      event "Test Name": Mouse Enter {
        # "Populate the ring with the list of tests"
        n198 = event-data() -> ()  [unwired: 1 in, 1 out]
        n199 = call <vilib>:"NT Read String Array.vi"("Name"="/TestMode/TestList") -> ("String Array"=w325:string[])  [unwired: 9 in, 1 out]
        n200 = Build Array (concatenate)("Select the test to run...", w325) -> (w324:string[])
        n201 = property on="Test Name" class="Ring (strict)"("Strings []"=w324) -> ()  [unwired: 2 in, 2 out]
      }
      event "Test Name": Value Change {
        w328 = FALSE ("Visible")
        # "Tell the robot the test name to run"
        n202 = event-data() -> ("NewVal"=w332:u16)  [unwired: 1 in]
        n203 = property on="Test Name" class="Ring (strict)"() -> ("Strings []"=w333:string[])  [unwired: 2 in, 2 out]
        n204 = local write "Progress"(T7 {"Test Progress"=0, "Test Progress Text"=""} ("Progress")) -> ()
        n205 = Index Array(array=w333, index=w332) -> (element=w331:string)
        n206 = call <vilib>:"NT Write String.vi"("String"=w331, "Name"="/TestMode/TestName") -> ()  [unwired: 9 in, 1 out]
        n207 = property on="Progress" class="Clust (strict)"("Visible"=TRUE) -> ()  [unwired: 2 in, 2 out]
        n208 = property on="Motor" class="Clust (strict)"("Visible"=w328) -> ()  [unwired: 2 in, 2 out]
        n209 = property on="Test Slider" class="Slide (strict)"("Visible"=w328) -> ()  [unwired: 2 in, 2 out]
        n210 = property on="On/Off" class="Bool (strict)"("Visible"=w328) -> ()  [unwired: 2 in, 2 out]
        n211 = property on="Rev/Fwd" class="Clust (strict)"("Visible"=w328) -> ()  [unwired: 2 in, 2 out]
        n212 = property on="Test Ring" class="Ring (strict)"("Visible"=w328) -> ()  [unwired: 2 in, 2 out]
      }
      event "Select Auto": Mouse Enter {
        # "Populate the combo box with the list of autonomous options"
        n213 = event-data() -> ()  [unwired: 1 in, 1 out]
        n214 = call <vilib>:"NT Read String Array.vi"("Name"="Auto List") -> ("String Array"=w335:string[])  [unwired: 9 in, 1 out]
        n215 = property on="Select Auto" class="CmbBox"("Strings[]"=w335) -> ()  [unwired: 2 in, 2 out]
      }
      event "Select Auto": Value Change {
        # "User modified the Auto Selection. Write to NT variable so robot knows."
        n216 = event-data() -> ("NewVal"=w339:string)  [unwired: 1 in]
        n217 = call <vilib>:"NT Write String.vi"("String"=w339, "Name"="Auto Selector") -> ()  [unwired: 9 in, 1 out]
      }
      event "Command Selection": Value Change {
        # "Get the params and show in table"
        n218 = event-data() -> ("NewVal"=w346:i32)  [unwired: 1 in]
        n219 = property on="Command Selection" class="MCListbox (strict)"() -> ("ItemNames"=w344:string[][])  [unwired: 2 in, 2 out]
        n220 = call <vilib>:"WPI_DashboardUpdate Command Params.vi"("NewVal"=w346, "Commands"=w344, "Param Tbl"=w345) -> ()  [unwired: 8 in, 1 out]
      }
      event "Execute Command": Value Change {
        # "Started one, Unique ID holds\nresponse"
        n221 = event-data() -> ()  [unwired: 1 in, 1 out]
        n222 = property on="Command Selection" class="MCListbox (strict)"() -> ("ItemNames"=w358:string[][])  [unwired: 2 in, 2 out]
        n223 = Index Array(array=w358, index (row)="Command Selection", index (col)=0) -> (element=w356:string)
        n224 = call <vilib>:"Invoke Commands.vi"("Command Params"="Command Params", "Function Name"=w356) -> ("Params"=w352:u8, "Started"=w351:bool)  [unwired: 7 in, 1 out]
        n225 = Array Subset(array="Command Params", length (row)=w352) -> (w353:string[][])  [unwired: 3 in]
        n226 = Select(t="Executing" ("Cmd Status"), s=w351, f="" ("Cmd Status")) -> (s? t:f=→"Cmd Status":string)
      }
      event "Command Selection": Double Click {
        n227 = event-data() -> ("Row"=w368:i32)  [unwired: 1 in]
        n228 = property on="Command Selection" class="MCListbox (strict)"() -> ("ItemNames"=w371:string[][])  [unwired: 2 in, 2 out]
        n229 = local read "Command Params"() -> (w366:string[][])
        n230 = Index Array(array=w371, index (row)=w368, index (col)=0) -> (element=w369:string)
        n231 = call <vilib>:"Invoke Commands.vi"("Command Params"=w366, "Function Name"=w369) -> ("Params"=w365:u8, "Started"=w360:bool)  [unwired: 7 in, 1 out]
        n232 = Array Subset(array=w366, length (row)=w365) -> (w364:string[][])  [unwired: 3 in]
        n233 = Select(t="Executing" ("Cmd Status"), s=w360, f="" ("Cmd Status")) -> (s? t:f=w361:string)
        n234 = local write "Cmd Status"(w361) -> ()
      }
      event "CheckList": Double Click {
        # "Shift clears all"
        # "Update symbols on the listbox"
        n235 = event-data() -> ("PlatMods.Shift"=w374:bool, "Row"=w376:i32)  [unwired: 1 in]
        n236 = case shown="True" w374 {
          tunnel: w376 -> [w380 _]
          tunnel: 1 -> [w379 _]
          frame False {
            n237 = property on="CheckList" class="LstBox (strict)"() -> ("Item Symbols"=w378:i32[])  [unwired: 2 in, 2 out]
            n238 = Replace Array Subset(array=w378, new element=w379, index=w380) -> (w377:i32[])
            n239 = property on="CheckList" class="LstBox (strict)"("Item Symbols"=w377) -> ()  [unwired: 2 in, 2 out]
          }
          frame True {
            w381 = 0 ("Top Row")
            n240 = property on="CheckList" class="LstBox (strict)"() -> ("Number of Rows"=w383:u32)  [unwired: 2 in, 2 out]
            n241 = Initialize Array(0, w383) -> (w382:i32[])
            n242 = property on="CheckList" class="LstBox (strict)"("Top Row"=w381, "Value"=w381, "Item Symbols"=w382) -> ()  [unwired: 2 in, 2 out]
          }
        }
      }
      event "CheckList": Key Down {
        # "Update symbols on the listbox\nLeft and right keys check and uncheck"
        n243 = event-data() -> ("VKey"=w388:T22)  [unwired: 1 in]
        n244 = case shown="\"Left\", \"Right\"" w388 {
          selector: w388 -> [w393 _]
          tunnel: eventvkey."Left" ("VKey") -> [w391 _]
          frame "Left", "Right" {
            n245 = Equal?(x=w391, y=w393) -> (x = y?=w392:bool)
            n246 = Select(t=0, s=w392, f=1) -> (s? t:f=w394:i32)
            n247 = property on="CheckList" class="LstBox (strict)"() -> ("Item Symbols"=w397:i32[])  [unwired: 2 in, 2 out]
            n248 = Replace Array Subset(array=w397, new element=w394, index="CheckList") -> (w396:i32[])
            n249 = property on="CheckList" class="LstBox (strict)"("Item Symbols"=w396) -> ()  [unwired: 2 in, 2 out]
          }
          frame Default {
          }
        }
      }
      event "DB Camera Config": Value Change {
        # "Show or hide the cluster of controls, store in ini file"
        n250 = event-data() -> ("NewVal"=w402:bool)  [unwired: 1 in]
        n251 = case shown="False" w402 {
          tunnel: w401 -> [w411 _]
          tunnel: [w404 w422] -> w400
          tunnel: w399 -> [w403 w422]
          frame False {
            w418 = "Camera"
            w421 = FALSE ("Visible")
            n252 = local read "Camera Settings"() -> (w410:T2)
            n253 = Index Array(array=w411) -> (element=w414:cluster{string[]})  [unwired: 1 in]
            n254 = Unbundle(w410) -> ("Frame Rate"=w409:i32, "Compression"=w408:i32, "Size"=w412:u16)
            n255 = Unbundle(w414) -> (w413:string[])
            n256 = Index Array(array=w413, index=w412) -> (element=w407:string)
            n257 = call-poly <vilib>:"Write Key.vi"("section"=w418, "value"=w407, "key"="Size", "refnum"=w403) -> ("refnum out"=w420:T20)  [unwired: 2 in, 5 out]
            n258 = call-poly <vilib>:"Write Key.vi"("section"=w418, "value"=w409, "key"="FrameRate", "refnum"=w420) -> ("refnum out"=w419:T20)  [unwired: 1 in, 6 out]
            n259 = property on="Camera Settings" class="Clust (strict)"("Visible"=w421) -> ()  [unwired: 2 in, 2 out]
            n260 = local write "DB Camera Config"(w421) -> ()
            n261 = call-poly <vilib>:"Write Key.vi"("section"=w418, "value"=w408, "key"="Compression", "refnum"=w419) -> ("refnum out"=w405:T20)  [unwired: 1 in, 6 out]
            n262 = call <vilib>:"Close Config Data.vi"("refnum"=w405) -> ("file path"=w406:path)  [unwired: 2 in, 8 out]
            n263 = call <vilib>:"Open Config Data.vi"("configuration file path"=w406) -> ("refnum"=w404:T20)  [unwired: 8 in, 2 out]
          }
          frame True {
            n264 = property on="Camera Settings" class="Clust (strict)"("Visible"=TRUE) -> ()  [unwired: 2 in, 2 out]
          }
        }
      }
      event "Camera Settings": Value Change {
        # "Update summary string when any elements of DB camera change"
        n265 = event-data() -> ("NewVal"=w436:T2)  [unwired: 1 in]
        n266 = Index Array(array=w432) -> (element=w431:cluster{string[]})  [unwired: 1 in]
        n267 = Unbundle(w436) -> ("Frame Rate"=w427:i32, "Compression"=w426:i32, "Size"=w429:u16)
        n268 = Unbundle(w431) -> (w430:string[])
        n269 = Index Array(array=w430, index=w429) -> (element=w428:string)
        n270 = Format Into String(format string="%s   %dfps   %d%%", w428, w427, w426) -> (resulting string=w433:string)  [unwired: 2 in, 1 out]
        n271 = Build Array(w433) -> (w434:string[])
        n272 = property on="DB Camera Config" class="Bool (strict)"("Strings [4]"=w434) -> ()  [unwired: 2 in, 2 out]
      }
      event "Motor.Enable": Value Change {
        # "When the test mode otor enable helper is set, update that\ntree row item's value"
        n273 = event-data() -> ("NewVal"=w443:bool)  [unwired: 1 in]
        n274 = Unbundle("Motor") -> ("Value"=w442:dbl)  [unwired: 1 out]
        n275 = Select(t=w442, s=w443, f=0.0) -> (s? t:f=w440:dbl)
        n276 = call <vilib>:"NT Write Number.vi"("Numeric"=w440, "Name"=w439) -> ()  [unwired: 9 in, 1 out]
      }
      event "Test Slider": Value Change {
        # "When the test mode slider helper is set, update that\ntree row item's value"
        n277 = event-data() -> ("NewVal"=w447:dbl)  [unwired: 1 in]
        n278 = call <vilib>:"NT Write Number.vi"("Numeric"=w447, "Name"=w448) -> ()  [unwired: 9 in, 1 out]
      }
      event "On/Off": Value Change {
        # "When the test mode on/off helper value is set, update that\ntree row item's value"
        n279 = event-data() -> ("NewVal"=w453:bool)  [unwired: 1 in]
        n280 = Boolean To (0,1)(Boolean=w453) -> (0, 1=w452:i16)
        n281 = call <vilib>:"NT Write Number.vi"("Numeric"=w452, "Name"=w451) -> ()  [unwired: 9 in, 1 out]
      }
      event "Rev/Fwd": Value Change {
        # "When the test mode helper value for relays is set, update that\ntree row item's value"
        n282 = event-data() -> ("NewVal.Forward"=w462:bool, "NewVal.Reverse"=w461:bool)  [unwired: 1 in]
        n283 = Boolean To (0,1)(Boolean=w462) -> (0, 1=w458:i16)
        n284 = Boolean To (0,1)(Boolean=w461) -> (0, 1=w460:i16)
        n285 = Negate(x=w460) -> (-x=w459:i16)
        n286 = Add(x=w458, y=w459) -> (x+y=w457:i16)
        n287 = call <vilib>:"NT Write Number.vi"("Numeric"=w457, "Name"=w456) -> ()  [unwired: 9 in, 1 out]
      }
      event "Test Ring": Value Change {
        # "When a test mode helper value is selected from the ring,\nset the tree item's variable to the string value"
        n288 = event-data() -> ("NewVal"=w467:u16)  [unwired: 1 in]
        n289 = property on="Test Ring" class="Ring (strict)"() -> ("Strings []"=w468:string[])  [unwired: 2 in, 2 out]
        n290 = Index Array(array=w468, index=w467) -> (element=w466:string)
        n291 = call <vilib>:"NT Write String.vi"("String"=w466, "Name"=w465) -> ()  [unwired: 9 in, 1 out]
      }
      event "Rec Mode": Value Change {
        # "Update globals for recording mode and path to read log from.\nClear when logging and let NetworkTables set path for vision to\nuse."
        n292 = event-data() -> ("NewVal"=w480:enum32{"Stop", "Record", "Playback"})  [unwired: 1 in]
        n293 = global write "WPI_DashboardLogging Global.vi" "Logging Filename"(path "") -> ()
        n294 = global write "WPI_DashboardLogging Global.vi" "Recording"(w480) -> ()
        n295 = case shown="\"Playback\"" w480 {
          tunnel: w479 -> [_ w482 w491]
          tunnel: [_ _ w490] -> w476
          tunnel: [_ _ w489] -> _
          tunnel: w474 -> [_ _ w487]
          tunnel: cluster{i32, i32} {-250, 170} -> [_ _ w486]
          tunnel: [_ _ T23 {"Image Size"=TRUE, "Image Type"=TRUE, "Pixel Value"=TRUE, "ROI Information"=TRUE, "Zoom Factor"=FALSE} ("Image Information Shown:All Elements")] -> w472
          tunnel: [_ _ TRUE ("Zoom Factor")] -> w471
          tunnel: w470 -> [_ _ w483]
          frame Default {
          }
          frame "Stop", "Record" {
            # "Place Window too"
            n296 = invoke class="VI" method="FP.Close"(reference=w482) -> (reference out=w481:refnum<vi>)  [unwired: 2 in, 2 out]
            n297 = invoke class="VI" method="Abort VI"(reference=w481) -> ()  [unwired: 2 in, 3 out]
          }
          frame "Playback" {
            n298 = call "Open Playback Panel.vi"("Offset"=w486, "DB VI Ref"=w487, "Playback in"=w491) -> ("Playback out"=w488:refnum<vi>)  [unwired: 8 in]
            n299 = register-events(w488, w483) -> (reference out=w490:refnum<event-registration>, error out=w489:errorcluster)  [unwired: 2 in]
          }
        }
        n300 = property on="Camera Image" class="ImageControl"("Image Information Shown"=w472, "Image Information Visible"=w471) -> ()  [unwired: 2 in, 2 out]
        n301 = call <vilib>:"WPI_DashboardNT Log FieldName Cache.vi"("Operation"=enum16{"Lookup/Add", "Index", "Clear"}."Clear") -> ()  [unwired: 8 in, 3 out]
      }
      event Panel Close {
        w493 = enum32{"Stop", "Record", "Playback"}."Stop" ("Rec Mode")
        # "Playback window has been closed, abort"
        n302 = event-data() -> ()  [unwired: 1 in, 4 out]
        n303 = local write "Rec Mode"(w493) -> ()
        n304 = global write "WPI_DashboardLogging Global.vi" "Recording"(w493) -> ()
      }
      event Panel Close {
        # "Abort playback window and ourself"
        n305 = event-data() -> ()  [unwired: 1 in, 4 out]
        n306 = invoke class="VI" method="FP.Close"(reference=w499) -> (reference out=w498:refnum<vi>)  [unwired: 2 in, 2 out]
        n307 = invoke class="VI" method="Abort VI"(reference=w498) -> (error out=w497:errorcluster)  [unwired: 2 in, 2 out]
        n308 = invoke class="VI" method="Abort VI"(error in=w497) -> ()  [unwired: 2 in, 3 out]
      }
      event User Event {
        n309 = event-data() -> ("IDs"=w507:cluster{"RPC field ID":u16, "Unique ID":u16}, "String"=w506:string)  [unwired: 1 in]
        n310 = Bundle("IDs"=w507, "String"=w506) -> (w505:T9)  [unwired: 1 in]
        n311 = call <vilib>:"Retrieve RPC Response.vi"("RPC Response"=w505) -> ("Output"=w502:string[][])  [unwired: 10 in]
        n312 = Build Array (concatenate)(w500, w502) -> (w501:string[][])
        n313 = local write "Command Params"(w501) -> ()
        n314 = local write "Cmd Status"("" ("Cmd Status")) -> ()
      }
      event "Vision": Value Change {
        # "Enable/Disable Compression slider.\nHW USB is hard-coded into the camera"
        n315 = event-data() -> ("NewVal"=w514:u16)  [unwired: 1 in]
        n316 = Equal?(x=w514, y=u32 2 ("milliseconds to wait")) -> (x = y?=w512:bool)
        n317 = Select(t=T24."Disabled and Grayed Out" ("Disabled"), s=w512, f=T24."Enabled" ("Disabled")) -> (s? t:f=w509:T24)
        n318 = property on="Compression" class="Slide (strict)"("DisabledEnum"=w509) -> ()  [unwired: 2 in, 2 out]
      }
      event "Tree": Double Click {
        n319 = event-data() -> ("PlatMods"=w519:T27, "Tag"=w518:string)  [unwired: 1 in]
        n320 = Unbundle(w519) -> ("Shift"=w517:bool)  [unwired: 4 out]
        n321 = Not(x=w517) -> (.not. x?=w516:bool)
        n322 = call <vilib>:"NT Update Persistence.vi"("Persistence"=w516, "Name"=w518) -> ()  [unwired: 9 in, 1 out]
      }
    }
  }
  n323 = while {
    tunnel: w47 -> [w523]
    i -> [w526]
    stop <- FALSE stop-if-true
    n324 = Wait (ms)(milliseconds to wait=u32 100) -> ()  [unwired: 1 out]
    n325 = case shown="\"Playback\"" "Rec Mode" {
      tunnel: w526 -> [_ _ w541]
      tunnel: [u32 2829099 ("Base Color") u32 11141120 ("Target Color") w530] -> w522
      frame "Stop", Default {
        # "Reset the color, extra updates don't cost much"
      }
      frame "Record" {
      }
      frame "Playback" {
        # "Playback"
        n326 = Quotient & Remainder(x=w541, y=u32 50 ("milliseconds to wait")) -> (x-y*floor(x/y)=w537:u32)  [unwired: 1 out]
        n327 = Divide(x=w537, y=u32 50 ("milliseconds to wait")) -> (x/y=w534:dbl)
        n328 = Multiply(x=6.283185307179586, y=w534) -> (x*y=w539:dbl)
        n329 = Sine(x=w539) -> (sin(x)=w538:dbl)
        n330 = Absolute Value(x=w538) -> (abs(x)=w531:dbl)
        n331 = call "Interpolate RGB Color.vi"("Proportion"=w531, "Target Color"=u32 30976, "Base Color"=u32 2829099) -> ("Result Color"=w530:u32)  [unwired: 8 in]
      }
    }
    n332 = property class="Pane"(reference=w523, "PaneColor"=w522) -> ()  [unwired: 1 in, 2 out]
  }
  n333 = local write "Dashboard Tab"(T1."Drive" ("Dashboard Tab")) -> ()
  n334 = property on="On/Off" class="Bool (strict)"("Visible"=w15) -> ()  [unwired: 2 in, 2 out]
  n335 = property on="Motor" class="Clust (strict)"("Visible"=w15) -> ()  [unwired: 2 in, 2 out]
  n336 = property on="Progress" class="Clust (strict)"("Visible"=w15) -> ()  [unwired: 2 in, 2 out]
  n337 = property on="Test Ring" class="Ring (strict)"("Visible"=w15) -> ()  [unwired: 2 in, 2 out]
  n338 = property on="Rev/Fwd" class="Clust (strict)"("Visible"=w15) -> ()  [unwired: 2 in, 2 out]
  n339 = property on="Camera Settings" class="Clust (strict)"("Visible"=w15) -> ()  [unwired: 2 in, 2 out]
  n340 = while {
    tunnel: u16 1741 ("timeout ms (25000)") -> [w543]
    stop <- FALSE stop-if-true
    n341 = TCP Create Listener(10:w543) -> (0:w542:errorcluster, 3:w544:refnum<k5>)  [unwired: 4 in, 1 out]
    n342 = case shown="No Error" w542 {
      selector: w542 -> [w546 _]
      tunnel: w544 -> [w547 _]
      frame No Error {
        n343 = while {
          tunnel: w547 -> [w550]
          tunnel: w546 -> [w549]
          stop <- FALSE stop-if-true
          n344 = TCP Wait On Listener(8:w549, 11:w550) -> (0:w551:errorcluster, 4:w552:refnum<k5>)  [unwired: 2 in, 3 out]
          n345 = local write "TCP"(w552) -> ()
          n346 = case shown="No Error" w551 {
            frame No Error {
            }
            frame Error {
              n347 = Wait (ms)(milliseconds to wait=u32 1000) -> ()  [unwired: 1 out]
            }
          }
        }
      }
      frame Error {
        n348 = Wait (ms)(milliseconds to wait=u32 1000) -> ()  [unwired: 1 out]
      }
    }
  }
  n349 = local write "DB Camera Config"(w15) -> ()
  n350 = local write "Command Params"(string[][] [] ("Command Params")) -> ()
  n351 = global write "WPI_DashboardLogging Global.vi" "Recording"(w41) -> ()
  n352 = local write "Command Selection"(u16 0 ("milliseconds to wait")) -> ()
  n353 = local write "Rec Mode"(w41) -> ()
